vi "SortNames.vi"(11 "Selected Paths":path[](array[path])) -> (3 "Selected Paths out":path[](array[path]))   [LabVIEW 2022 SP3]
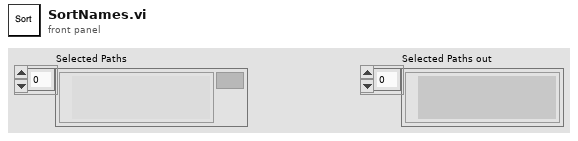
[diagram p1: front panel]
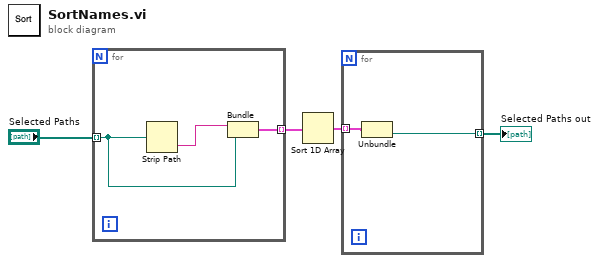
[diagram p0: block diagram]
diagram:
  n1 = for {
    tunnel: "Selected Paths" -> [w7] mode=indexing
    tunnel: [w6] -> w3 mode=indexing
    n2 = Strip Path(path=w7) -> (name=w5:string)  [unwired: 1 out]
    n3 = Bundle("name"=w5, "selected path"=w7) -> (w6:cluster{"name":string, "selected path":path})  [unwired: 1 in]
  }
  n4 = Sort 1D Array(array=w3) -> (sorted array=w2:cluster{"name":string, "selected path":path}[])
  n5 = for {
    tunnel: w2 -> [w9] mode=indexing
    tunnel: [w8] -> w1 mode=indexing
    n6 = Unbundle(w9) -> ("selected path"=w8:path)  [unwired: 1 out]
  }
  "Selected Paths out" <- w1
